vi "Read TopRow.vi"(8 "error in (no error)":errorcluster, 11 "BetterMultiListboxHandle in":refnum<class "BetterMultiListboxHandle.lvclass">) -> (0 "error out":errorcluster, 2 "TopRow":i32, 3 "BetterMultiListboxHandle out":refnum<class "BetterMultiListboxHandle.lvclass">)   [LabVIEW 2020, in "BetterDragAndDrop.lvlib" / "BetterMultiListboxHandle.lvclass"]
uses:
  BetterMultiListboxHandle.lvclass
  BetterMultiListboxHandle.lvclass/BetterMultiListboxHandle.ctl
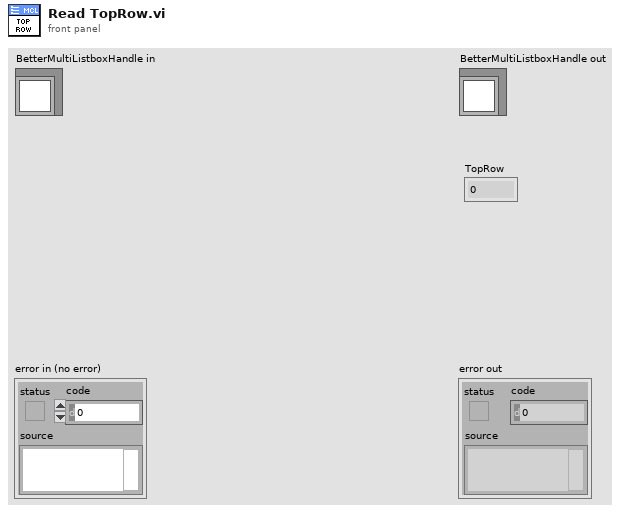
[diagram p1: front panel]
types:
  T1 = typedef "LVRowAndColumnUnsignedTypeDef.ctl" = cluster{"Row":u32, "Column":u32}
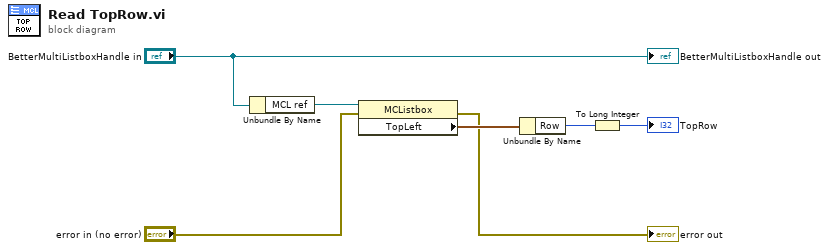
[diagram p0: block diagram]
diagram:
  n1 = Unbundle By Name("BetterMultiListboxHandle in") -> ("MCL ref"=w6:refnum<vi>)
  n2 = property class="MCListbox"(reference=w6, error in="error in (no error)") -> (error out=→"error out":errorcluster, "TopLeft"=w5:T1)  [unwired: 1 out]
  n3 = Unbundle By Name(w5) -> ("Row"=w4:u32)
  n4 = To Long Integer(number=w4) -> (32bit integer=→"TopRow":i32)
  "BetterMultiListboxHandle out" <- "BetterMultiListboxHandle in"
